vi "Configure Programmer Parameters (Program Off).vi"(7 "Unit Address (1)":u8=1, 8 "error in (no error)":errorcluster, 9 "Reset Event Outputs (0)":u8, 10 "Current Program Number (1)":u8=1 min=1 max=50, 11 "VISA resource name":refnum<visa-resource-name>) -> (0 "error out":errorcluster, 3 "VISA resource name out":refnum<visa-resource-name>)   [LabVIEW 2014, in "Eurotherm 35xx Series.lvlib"]
doc: "This VI sets Programmer Parameters in Program \"Off\" status."
uses:
  <instrlib>/Eurotherm 35xx Series/Eurotherm 35xx Series.lvlib
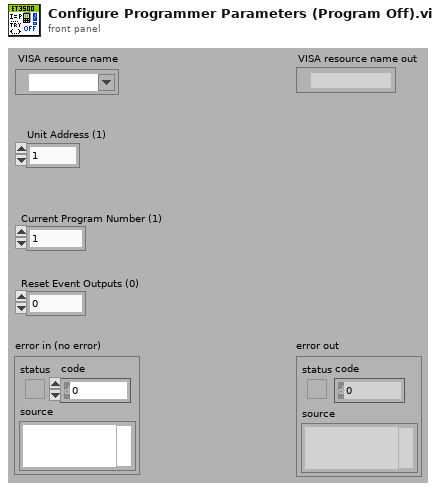
[diagram p1: front panel]
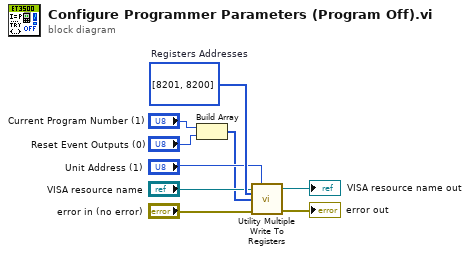
[diagram p0: block diagram]
diagram:
  w7 = u16[] [8201, 8200]  # Registers Addresses
  n1 = Build Array("Current Program Number (1)", "Reset Event Outputs (0)") -> (w1:u8[])
  n2 = call <instrlib>:"Utility Multiple Write To Registers.vi"("VISA resource name"="VISA resource name", "Unit Address (1)"="Unit Address (1)", "Registers Addresses (0)"=w7, "Data (0)"=w1, "error in (no error)"="error in (no error)") -> ("VISA resource name out"=→"VISA resource name out":refnum<visa-resource-name>, "error out"=→"error out":errorcluster)  [unwired: 9 in]
